vi "Stream data to voltages and currents.vi"(8 "Polarities":bool[](array[boolean]), 10 "Stream channels":string[][](array[string]), 11 "Stream data":dbl[][](array[numeric])) -> (3 "Data out":dbl[](array[numeric]))   [LabVIEW 2018]
uses:
  <vilib>/Analysis/baseanly.llb/Mean (DBL).vi
  <vilib>/Analysis/NI_AALBase.lvlib
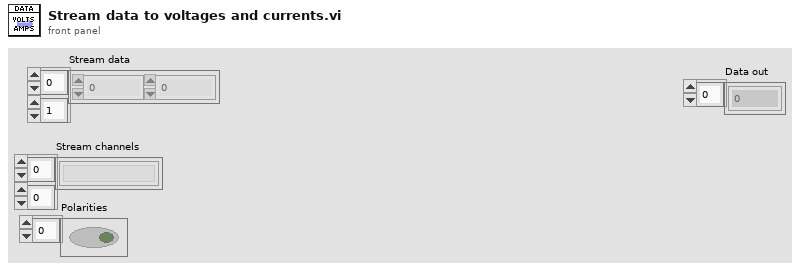
[diagram p1: front panel]
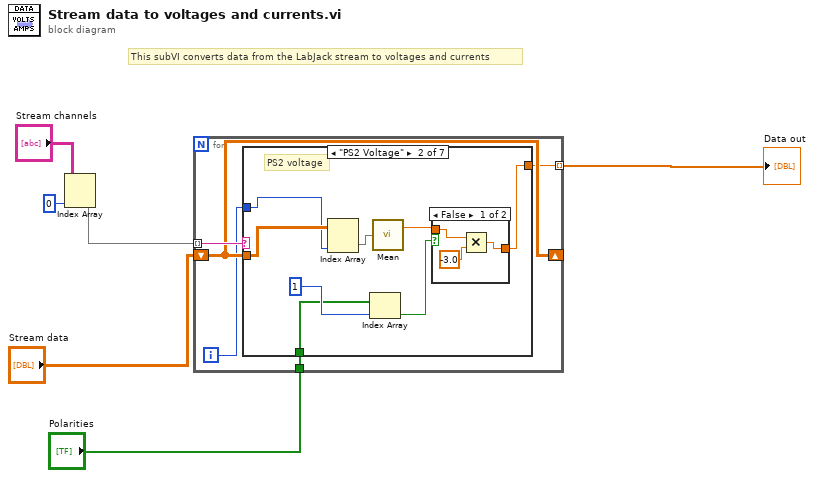
[diagram p0: block diagram]
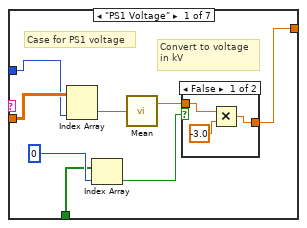
[diagram p2: hidden frame]
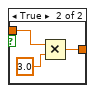
[diagram p3: hidden frame]
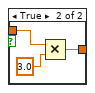
[diagram p4: hidden frame]
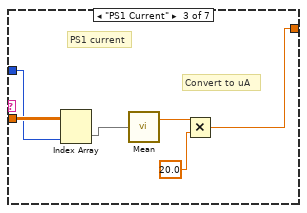
[diagram p5: hidden frame]
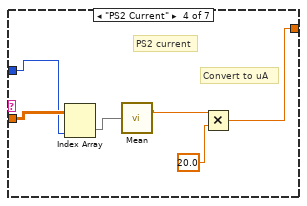
[diagram p6: hidden frame]
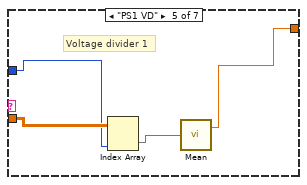
[diagram p7: hidden frame]
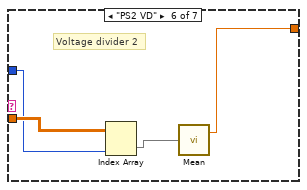
[diagram p8: hidden frame]
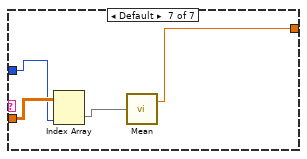
[diagram p9: hidden frame]
diagram:
  # "This subVI converts data from the LabJack stream to voltages and currents"
  n1 = Index Array(array="Stream channels", index (col)=0 ("disabled index (col)")) -> (element=w2:string[])  [unwired: 1 in]
  n2 = for {
    tunnel: w2 -> [w11] mode=indexing
    shift-right: [w10] -> _
    shift-left: "Stream data" -> [w10]
    tunnel: [w9] -> w4 mode=indexing
    tunnel: "Polarities" -> [w8]
    i -> [w7]
    n3 = case shown="\"PS2 Voltage\"" w11 {
      tunnel: w10 -> [w19 w33 w44 w50 w54 w57 w61]
      tunnel: [w16 w31 w42 w47 w53 w58 w62] -> w9
      tunnel: w8 -> [w14 w27 _ _ _ _ _]
      tunnel: w7 -> [w12 w26 w40 w46 w52 w56 w60]
      frame "PS1 Voltage" {
        # "Convert to voltage\nin kV"
        # "Case for PS1 voltage"
        n4 = Index Array(array=w19, index (col)=w12) -> (element=w18:dbl[])  [unwired: 1 in]
        n5 = Index Array(array=w14, index=0) -> (element=w13:bool)
        n6 = call-poly <vilib>:"Mean.vi"("X"=w18) -> ("mean"=w17:dbl)  [unwired: 1 out]
        n7 = case shown="False" w13 {
          tunnel: w17 -> [w21 w25]
          tunnel: [w20 w23] -> w16
          frame False {
            n8 = Multiply(x=w21, y=-3.0) -> (x*y=w20:dbl)
          }
          frame True {
            n9 = Multiply(x=w25, y=3.0) -> (x*y=w23:dbl)
          }
        }
      }
      frame "PS2 Voltage" {
        # "PS2 voltage"
        n10 = Index Array(array=w33, index (col)=w26) -> (element=w32:dbl[])  [unwired: 1 in]
        n11 = Index Array(array=w27, index=1) -> (element=w28:bool)
        n12 = call-poly <vilib>:"Mean.vi"("X"=w32) -> ("mean"=w30:dbl)  [unwired: 1 out]
        n13 = case shown="False" w28 {
          tunnel: w30 -> [w35 w39]
          tunnel: [w34 w37] -> w31
          frame False {
            n14 = Multiply(x=w35, y=-3.0) -> (x*y=w34:dbl)
          }
          frame True {
            n15 = Multiply(x=w39, y=3.0) -> (x*y=w37:dbl)
          }
        }
      }
      frame "PS1 Current" {
        # "Convert to uA"
        # "PS1 current"
        n16 = Index Array(array=w44, index (col)=w40) -> (element=w45:dbl[])  [unwired: 1 in]
        n17 = call-poly <vilib>:"Mean.vi"("X"=w45) -> ("mean"=w43:dbl)  [unwired: 1 out]
        n18 = Multiply(x=w43, y=20.0) -> (x*y=w42:dbl)
      }
      frame "PS2 Current" {
        # "Convert to uA"
        # "PS2 current"
        n19 = Index Array(array=w50, index (col)=w46) -> (element=w51:dbl[])  [unwired: 1 in]
        n20 = call-poly <vilib>:"Mean.vi"("X"=w51) -> ("mean"=w48:dbl)  [unwired: 1 out]
        n21 = Multiply(x=w48, y=20.0) -> (x*y=w47:dbl)
      }
      frame "PS1 VD" {
        # "Voltage divider 1"
        n22 = Index Array(array=w54, index (col)=w52) -> (element=w55:dbl[])  [unwired: 1 in]
        n23 = call-poly <vilib>:"Mean.vi"("X"=w55) -> ("mean"=w53:dbl)  [unwired: 1 out]
      }
      frame "PS2 VD" {
        # "Voltage divider 2"
        n24 = Index Array(array=w57, index (col)=w56) -> (element=w59:dbl[])  [unwired: 1 in]
        n25 = call-poly <vilib>:"Mean.vi"("X"=w59) -> ("mean"=w58:dbl)  [unwired: 1 out]
      }
      frame Default {
        n26 = Index Array(array=w61, index (col)=w60) -> (element=w63:dbl[])  [unwired: 1 in]
        n27 = call-poly <vilib>:"Mean.vi"("X"=w63) -> ("mean"=w62:dbl)  [unwired: 1 out]
      }
    }
  }
  "Data out" <- w4
